vi "xbee_command.vi"(8 "error in (no error)":errorcluster, 10 "command":string="+++", 11 "COM in":refnum<visa-resource-name>) -> (0 "error out":errorcluster, 2 "read buffer":string, 3 "COM out":refnum<visa-resource-name>)   [LabVIEW 2012]
uses:
  <vilib>/Instr/_visa.llb/VISA Configure Serial Port (Instr).vi
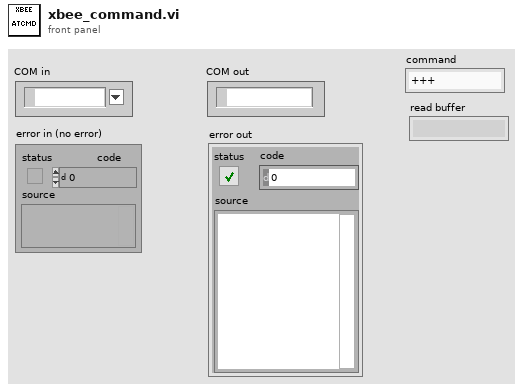
[diagram p1: front panel]
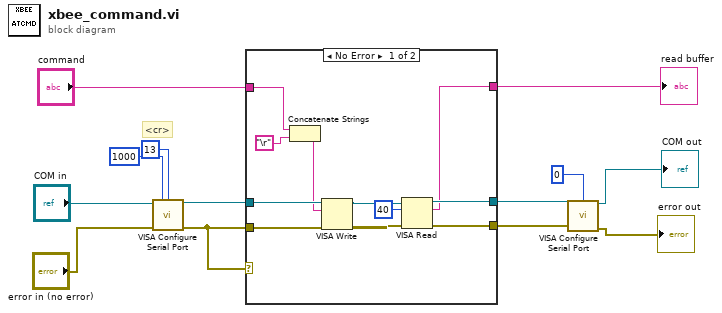
[diagram p0: block diagram]
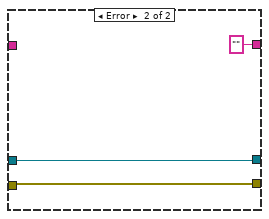
[diagram p2: hidden frame]
diagram:
  # "<cr>"
  n1 = call-poly "VISA Configure Serial Port"("VISA resource name"="COM in", "timeout (10sec)"=u32 1000, "termination char\n(0xA = '\\n' = LF)"=u8 13 ("termination char\n(0xA = '\\n' = LF)"), "error in (no error)"="error in (no error)") -> ("VISA resource name out"=w13:refnum<visa-resource-name>, "error out"=w12:errorcluster)  [unwired: 10 in]
  n2 = case shown="No Error" w12 {
    tunnel: w13 -> [w24 w27]
    tunnel: w12 -> [w23 w26]
    tunnel: [w18 w27] -> w3
    tunnel: [w19 w26] -> w2
    tunnel: "command" -> [w15 _]
    tunnel: [w17 "" ("read buffer")] -> w6
    frame No Error {
      n3 = Concatenate Strings(w15, "\r") -> (w14:string)
      n4 = VISA Write(VISA resource name=w24, write buffer=w14, error in (no error)=w23) -> (VISA resource name out=w20:refnum<visa-resource-name>, error out=w21:errorcluster)  [unwired: 1 out]
      n5 = VISA Read(VISA resource name=w20, byte count=u32 40, error in (no error)=w21) -> (VISA resource name out=w18:refnum<visa-resource-name>, read buffer=w17:string, error out=w19:errorcluster)  [unwired: 1 out]
    }
    frame Error {
    }
  }
  "read buffer" <- w6
  n6 = call-poly "VISA Configure Serial Port"("VISA resource name"=w3, "termination char\n(0xA = '\\n' = LF)"=u8 0 ("termination char\n(0xA = '\\n' = LF)"), "error in (no error)"=w2) -> ("VISA resource name out"=→"COM out":refnum<visa-resource-name>, "error out"=→"error out":errorcluster)  [unwired: 11 in]
